vi "New DVR VI.vi"(0 "Read DVR Value":bool, 11 "error in":errorcluster) -> (4 "DVR Value":dbl, 15 "error out":errorcluster)   [LabVIEW 2023]
doc: "New DVR VI receives the DVR reference from the DVR Creator VI and displays the incremented numeric double value when Read DVR Value boolean is pressed."
uses:
  LV2/Controls/LV2Operations.ctl
panel:
  # "INSTRUTIONS :\n\n1. Run the VI. \n2. Make sure the DVR Creator VI is running \n3. Press Read DVR Value button to receive the \n   incremented numeric value from the DVR \n   Creator VI.\n4. Panel close to abort th VI."
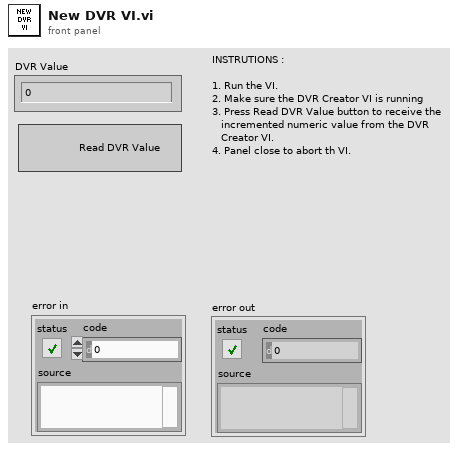
[diagram p1: front panel]
types:
  T1 = typedef "LV2Operations.ctl" = enum16{"Init", "Read", "Write"}
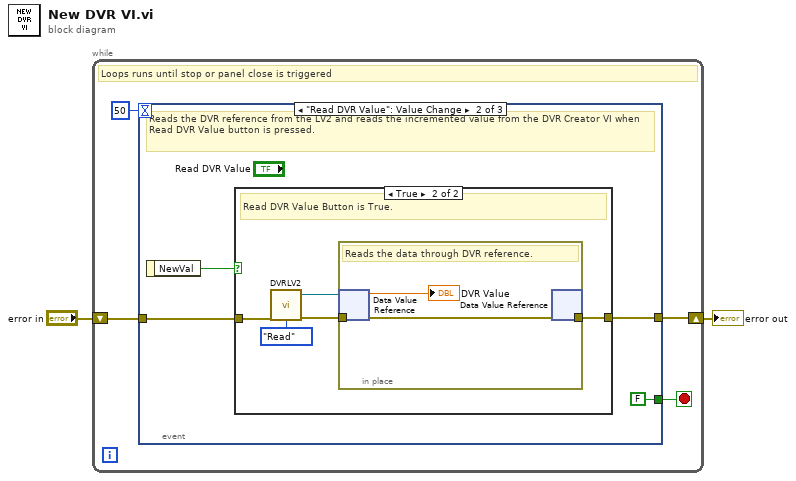
[diagram p0: block diagram]
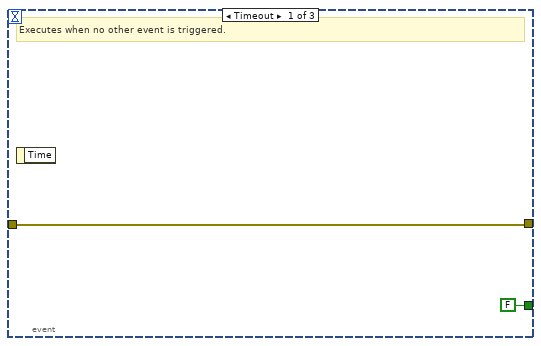
[diagram p2: hidden frame]
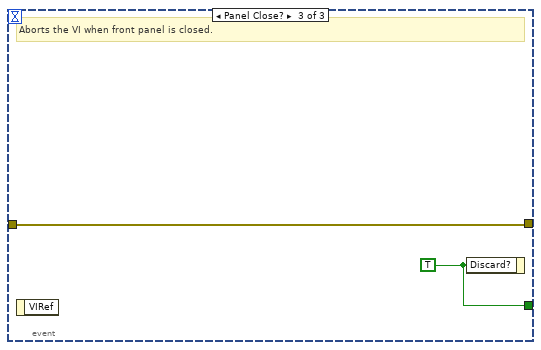
[diagram p4: hidden frame]
diagram:
  n1 = while {
    shift-right: [w3] -> w1
    shift-left: "error in" -> [w4]
    stop <- w5 stop-if-true
    # "Loops runs until stop or panel close is triggered"
    n2 = event shown="[1] \"Read DVR Value\": Value Change" {
      selector: _ -> [_ _ _]
      dyn-events: _ -> [_ _ _]
      timeout: 50 -> [_ _ _]
      tunnel: [FALSE ("Discard?") FALSE ("stop") w21] -> w5
      tunnel: w4 -> [w8 w10 w22]
      tunnel: [w8 w9 w22] -> w3
      event Timeout {
        # "Executes when no other event is triggered."
        n3 = event-data() -> ()  [unwired: 1 in, 1 out]
      }
      event "Read DVR Value": Value Change {
        # "Reads the DVR reference from the LV2 and reads the incremented value from the DVR Creator VI when Read DVR Value button is pressed."
        n4 = event-data() -> ("NewVal"=w11:bool)  [unwired: 1 in]
        n5 = case shown="True" w11 {
          tunnel: w10 -> [w13 w17]
          tunnel: [w13 w15] -> w9
          frame False {
            # "Read DVR Value Button is False."
          }
          frame True {
            # "Read DVR Value Button is True."
            n6 = call "DVRLV2.vi"("error in"=w17, "Operations"=LV2Operations."Read") -> ("data value reference out"=w16:refnum<data-value>, "error out"=w14:errorcluster)  [unwired: 12 in]
            n7 = in-place {
              in-place-border: w14 -> [_]
              in-place-border: [w19] -> _
              # "Reads the data through DVR reference."
              n8 = in-place-dvr #1(w16) -> (→"DVR Value":dbl, w19:errorcluster)
              n9 = in-place-dvr #1() -> (w15:errorcluster)  [unwired: 1 in, 1 out]
            }
          }
        }
      }
      event Panel Close? {
        w21 = TRUE ("Discard?")
        # "Aborts the VI when front panel is closed."
        n10 = event-data() -> ()  [unwired: 1 in, 1 out]
        n11 = event-data("Discard?"=w21) -> ()  [unwired: 1 in, 1 out]
      }
    }
  }
  "error out" <- w1
